vi "Initialize Buffer.vi"(0 "Session Handle in":T1, 5 "Size":u16, 11 "error in (no error)":errorcluster) -> (4 "Session Handle out":T1, 15 "error out":errorcluster)   [LabVIEW 2015, in "Circular Buffer.lvclass"]
uses:
  Circular Buffer.lvclass
  Typedefs/Session Handle.ctl
  Circular Buffer.lvclass/Circular Buffer.ctl
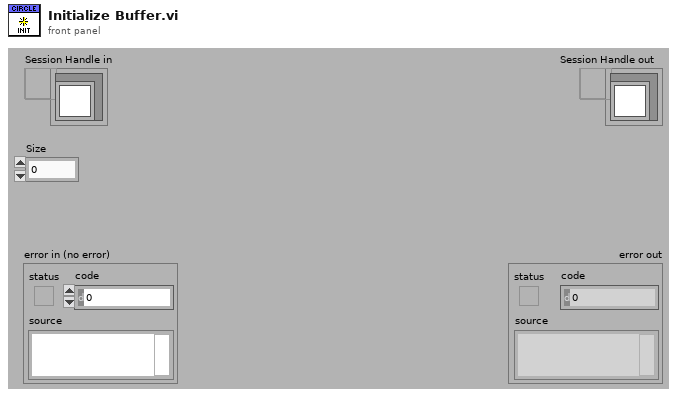
[diagram p1: front panel]
types:
  T1 = typedef "Circular Buffer.lvclass/Session Handle.ctl" = refnum<data-value>
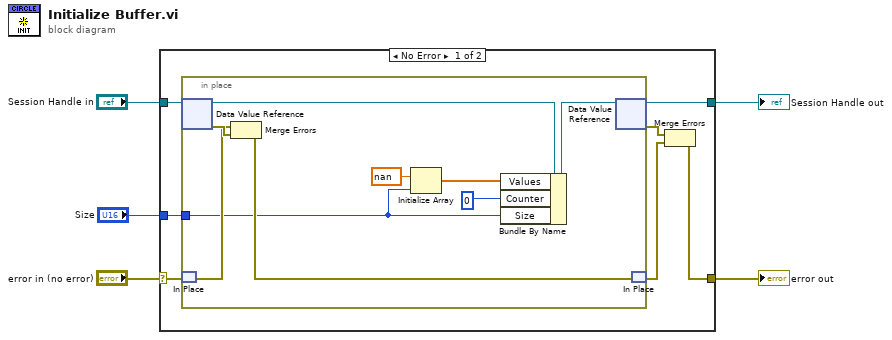
[diagram p0: block diagram]
diagram:
  n1 = case shown="No Error" "error in (no error)" {
    selector: "error in (no error)" -> [w7 w22]
    tunnel: "Session Handle in" -> [w12 w23]
    tunnel: [w11 w23] -> w4
    tunnel: [w8 w22] -> w3
    tunnel: "Size" -> [w6 _]
    frame No Error {
      n2 = in-place {
        in-place-border: w6 -> [w13]
        n3 = in-place-dvr #1(w12) -> (w15:refnum<class "Circular Buffer.lvclass">, w20:errorcluster)
        n4 = in-place-match #2(w7) -> (w19:errorcluster)
        n5 = Merge Errors(w19, w20) -> (w21:errorcluster)
        n6 = Initialize Array(nan ("element"), w13) -> (w17:dbl[])
        n7 = Bundle By Name(cluster=w15, "Values"=w17, "Counter"=u16 0, "Size"=w13) -> (w14:refnum<class "Circular Buffer.lvclass">)
        n8 = in-place-dvr #1(w14) -> (w11:T1, w9:errorcluster)
        n9 = in-place-match #2(w21) -> (w10:errorcluster)
      }
      n10 = Merge Errors(w9, w10) -> (w8:errorcluster)
    }
    frame Error {
    }
  }
  "Session Handle out" <- w4
  "error out" <- w3
